vi "总磷数据时间处理.vi"(9 "总磷修正数据输入":T1 {"单位" items=["ug/L", "mg/L", "ppm", "mg/m3", "cm", "ppb", "ug/m3", "%", "nmol/mol", "umol/mol", "MPN/L", "MPN/100ml", "ng/m3", "NTU", "无量纲", "ms/cm", "us/cm", "℃", "mV", "万个/L"]}, 10 "总氮原始数据":T1 {"单位" items=["ug/L", "mg/L", "ppm", "mg/m3", "cm", "ppb", "ug/m3", "%", "nmol/mol", "umol/mol", "MPN/L", "MPN/100ml", "ng/m3", "NTU", "无量纲", "ms/cm", "us/cm", "℃", "mV", "万个/L"]}, 11 "总磷原始数据":T1 {"单位" items=["ug/L", "mg/L", "ppm", "mg/m3", "cm", "ppb", "ug/m3", "%", "nmol/mol", "umol/mol", "MPN/L", "MPN/100ml", "ng/m3", "NTU", "无量纲", "ms/cm", "us/cm", "℃", "mV", "万个/L"]}) -> (3 "总磷修正数据输出":T1 {"单位" items=["ug/L", "mg/L", "ppm", "mg/m3", "cm", "ppb", "ug/m3", "%", "nmol/mol", "umol/mol", "MPN/L", "MPN/100ml", "ng/m3", "NTU", "无量纲", "ms/cm", "us/cm", "℃", "mV", "万个/L"]})   [LabVIEW 2016, in "斯坦道总氮.lvlib"]
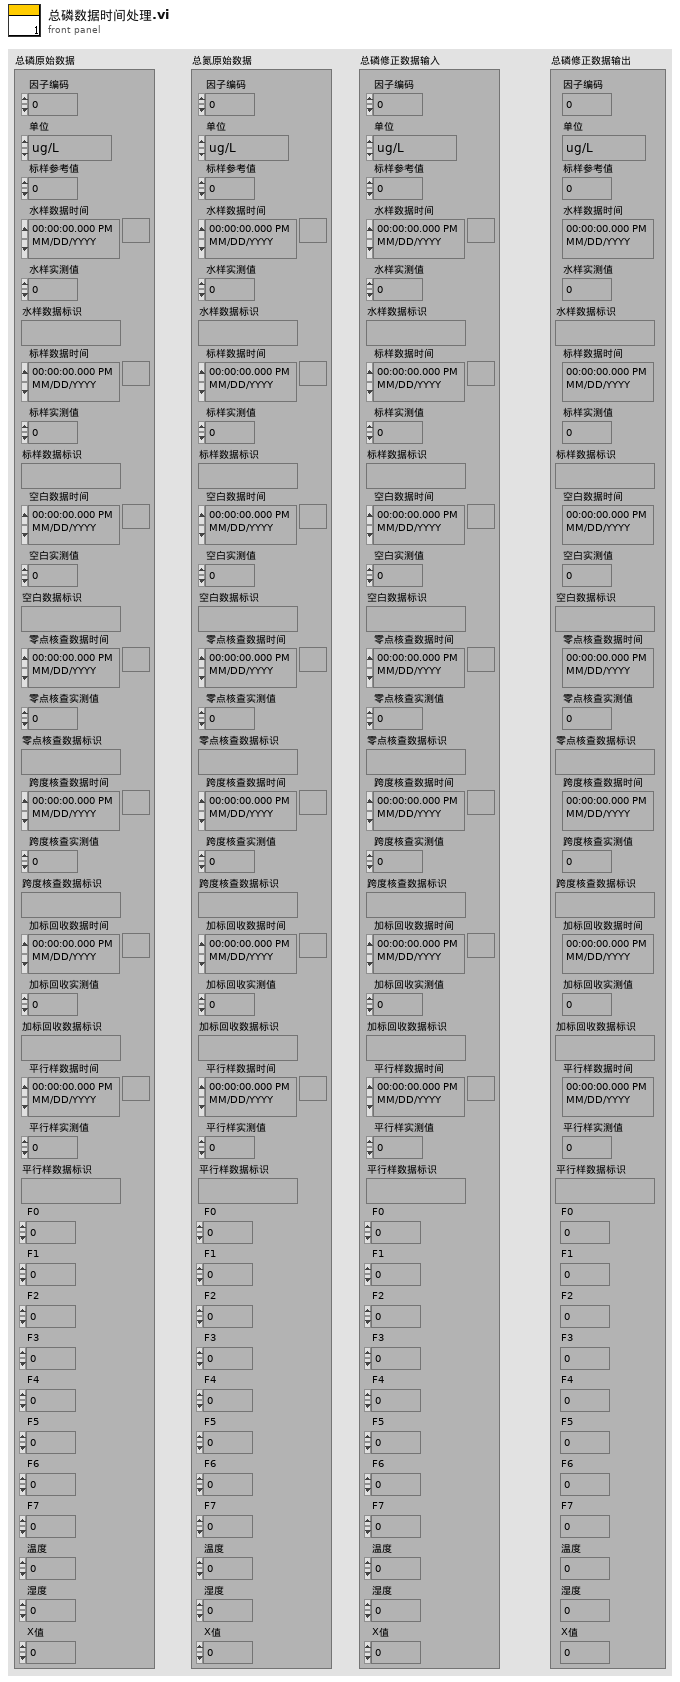
[diagram p1: front panel]
types:
  T1 = cluster{"因子编码":u32, "单位":u16, "标样参考值":sgl, "水样数据时间":timestamp, "水样实测值":sgl, "水样数据标识":string, "标样数据时间":timestamp, "标样实测值":sgl, "标样数据标识":string, "空白数据时间":timestamp, "空白实测值":sgl, "空白数据标识":string, "零点核查数据时间":timestamp, "零点核查实测值":sgl, "零点核查数据标识":string, "跨度核查数据时间":timestamp, "跨度核查实测值":sgl, "跨度核查数据标识":string, "加标回收数据时间":timestamp, "加标回收实测值":sgl, "加标回收数据标识":string, "平行样数据时间":timestamp, "平行样实测值":sgl, "平行样数据标识":string, "F0":sgl, "F1":sgl, "F2":sgl, "F3":sgl, "F4":sgl, "F5":sgl, "F6":sgl, "F7":sgl, "温度":sgl, "湿度":sgl, "X值":sgl}
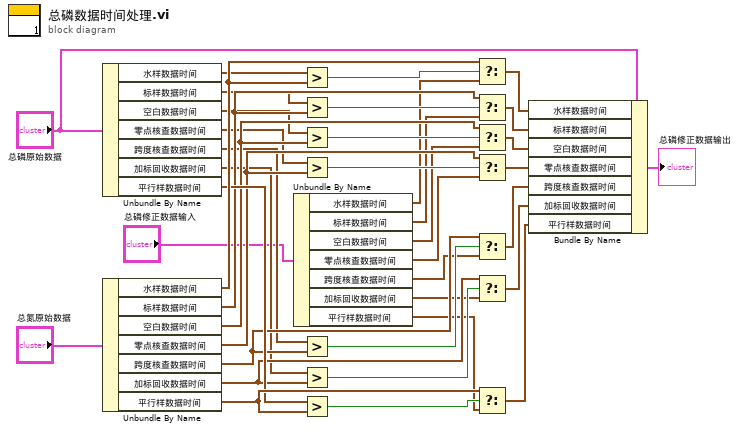
[diagram p0: block diagram]
diagram:
  n1 = Unbundle By Name("总磷原始数据") -> ("水样数据时间"=w34:timestamp, "标样数据时间"=w22:timestamp, "空白数据时间"=w19:timestamp, "零点核查数据时间"=w16:timestamp, "跨度核查数据时间"=w13:timestamp, "加标回收数据时间"=w9:timestamp, "平行样数据时间"=w30:timestamp)
  n2 = Unbundle By Name("总氮原始数据") -> ("水样数据时间"=w35:timestamp, "标样数据时间"=w23:timestamp, "空白数据时间"=w20:timestamp, "零点核查数据时间"=w17:timestamp, "跨度核查数据时间"=w14:timestamp, "加标回收数据时间"=w10:timestamp, "平行样数据时间"=w31:timestamp)
  n3 = Unbundle By Name("总磷修正数据输入") -> ("水样数据时间"=w7:timestamp, "标样数据时间"=w6:timestamp, "空白数据时间"=w5:timestamp, "零点核查数据时间"=w4:timestamp, "跨度核查数据时间"=w3:timestamp, "加标回收数据时间"=w2:timestamp, "平行样数据时间"=w1:timestamp)
  n4 = Greater?(x=w34, y=w35) -> (0:w36:bool)
  n5 = Greater?(x=w22, y=w23) -> (0:w24:bool)
  n6 = Greater?(x=w19, y=w20) -> (0:w25:bool)
  n7 = Greater?(x=w16, y=w17) -> (0:w26:bool)
  n8 = Greater?(x=w13, y=w14) -> (0:w27:bool)
  n9 = Greater?(x=w9, y=w10) -> (0:w28:bool)
  n10 = Greater?(x=w30, y=w31) -> (0:w32:bool)
  n11 = Select(t=w35, s=w36, f=w7) -> (s? t:f=w33:timestamp)
  n12 = Select(t=w23, s=w24, f=w6) -> (s? t:f=w21:timestamp)
  n13 = Select(t=w20, s=w25, f=w5) -> (s? t:f=w18:timestamp)
  n14 = Select(t=w17, s=w26, f=w4) -> (s? t:f=w15:timestamp)
  n15 = Select(t=w14, s=w27, f=w3) -> (s? t:f=w12:timestamp)
  n16 = Select(t=w10, s=w28, f=w2) -> (s? t:f=w11:timestamp)
  n17 = Select(t=w31, s=w32, f=w1) -> (s? t:f=w29:timestamp)
  n18 = Bundle By Name(cluster="总磷原始数据", "水样数据时间"=w33, "标样数据时间"=w21, "空白数据时间"=w18, "零点核查数据时间"=w15, "跨度核查数据时间"=w12, "加标回收数据时间"=w11, "平行样数据时间"=w29) -> (→"总磷修正数据输出":T1)
